vi "Node Names.vi"(11 "Module in":refnum<class "Module.lvclass">) -> (0 "Node":string, 1 "Cluster":string, 2 "System":string, 3 "Module out":refnum<class "Module.lvclass">, 4 "Node ID":u32)   [LabVIEW 2020, in "Volatus.lvlib" / "Module.lvclass"]
uses:
  Module.lvclass
  Module.lvclass/Module.ctl
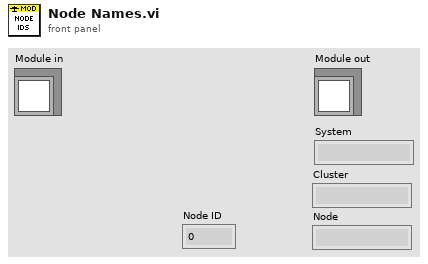
[diagram p1: front panel]
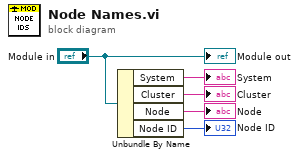
[diagram p0: block diagram]
diagram:
  n1 = Unbundle By Name("Module in") -> ("System"=→"System":string, "Cluster"=→"Cluster":string, "Node"=→"Node":string, "Node ID"=→"Node ID":u32)
  "Module out" <- "Module in"
